vi "MESParameter.vi"(8 "error in (no error)":errorcluster, 10 "MES Data":T1, 11 "Step":enum16{"Initial", "Write", "Read"}(ring)) -> (0 "error out":errorcluster, 3 "MES Data 2":T1)   [LabVIEW 2017]
uses:
  Ctrls/MES Data.ctl
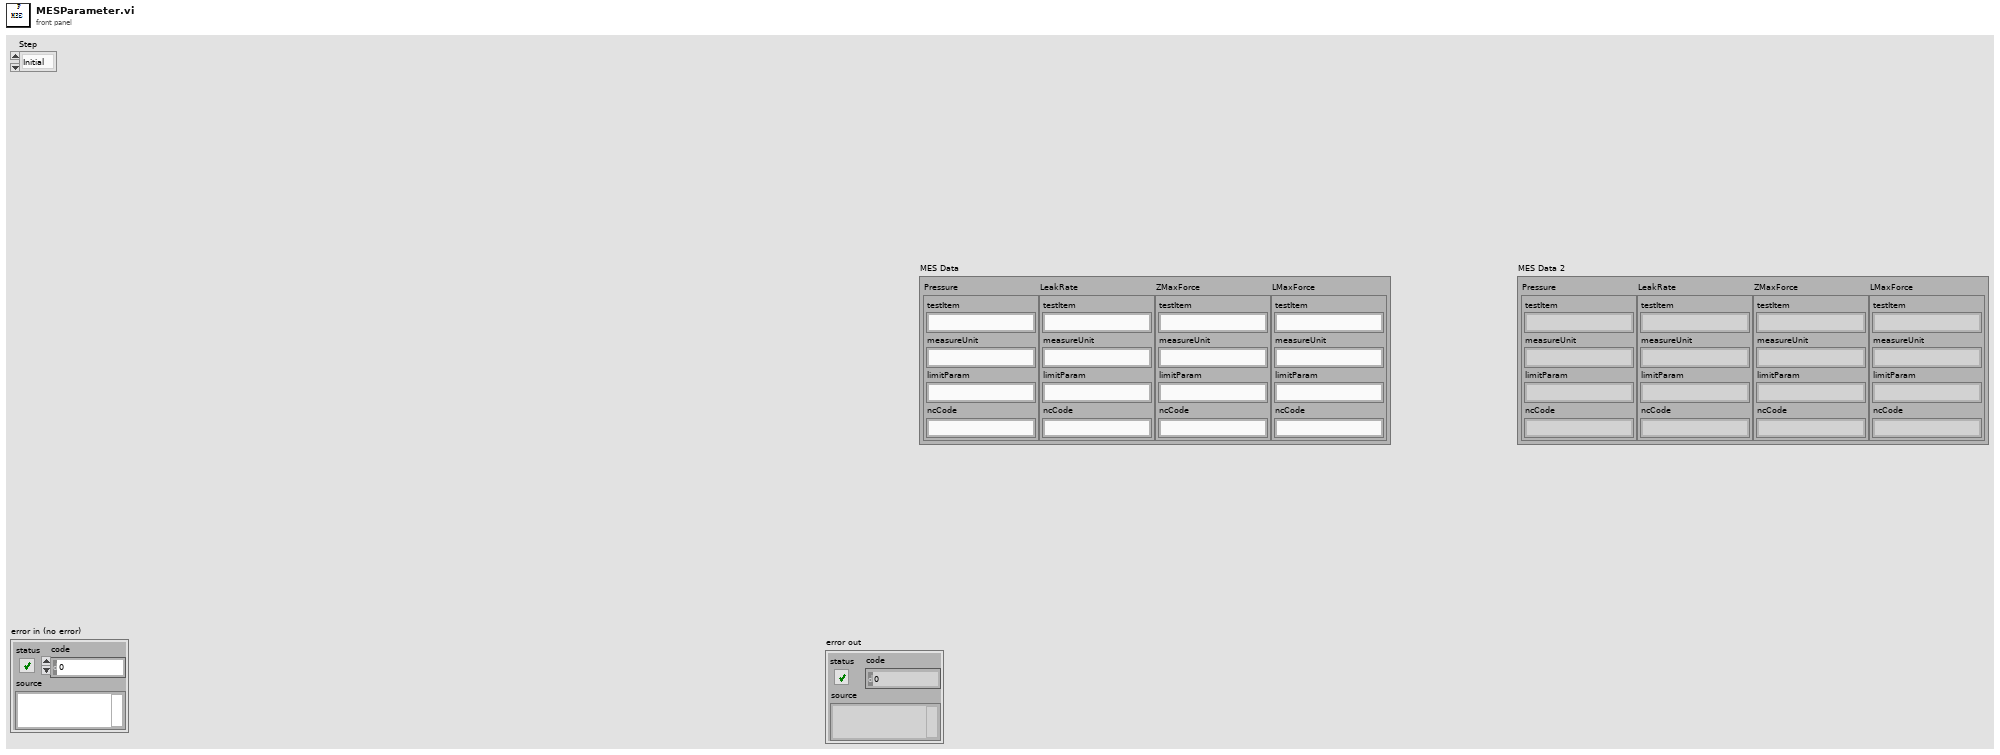
[diagram p1: front panel]
types:
  T1 = typedef "MES Data.ctl" = cluster{"Pressure":cluster{"testItem":string, "measureUnit":string, "limitParam":string, "ncCode":string}, "LeakRate":cluster{"testItem":string, "measureUnit":string, "limitParam":string, "ncCode":string}, "ZMaxForce":cluster{"testItem":string, "measureUnit":string, "limitParam":string, "ncCode":string}, "LMaxForce":cluster{"testItem":string, "measureUnit":string, "limitParam":string, "ncCode":string}}
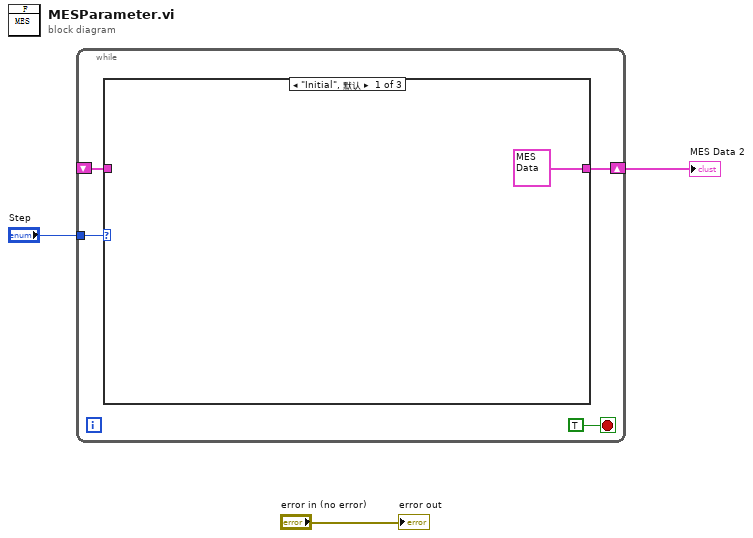
[diagram p0: block diagram]
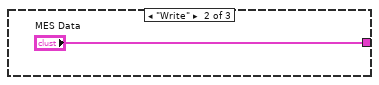
[diagram p2: hidden frame]
diagram:
  n1 = while {
    tunnel: "Step" -> [w6]
    shift-right: [w5] -> w1
    shift-left: _ -> [w4]
    stop <- TRUE stop-if-true
    n2 = case shown="\"Initial\", 默认" w6 {
      tunnel: [T1 {"Pressure"={"testItem"="", "measureUnit"="", "limitParam"="", "ncCode"=""}, "LeakRate"={"testItem"="", "measureUnit"="", "limitParam"="", "ncCode"=""}, "ZMaxForce"={"testItem"="", "measureUnit"="", "limitParam"="", "ncCode"=""}, "LMaxForce"={"testItem"="", "measureUnit"="", "limitParam"="", "ncCode"=""}} ("MES Data") "MES Data" w10] -> w5
      tunnel: w4 -> [_ _ w10]
      frame "Initial", Default {
      }
      frame "Write" {
      }
      frame "Read" {
      }
    }
  }
  "MES Data 2" <- w1
  "error out" <- "error in (no error)"
